vi "MainThang.vi"() -> ()   [LabVIEW 2020]
uses:
  TypeDefs/MainQueueEnumVariant.ctl
  TypeDefs/Item Cluster.ctl
panel:
  in  "Input Buttons":T1
  out "Diplay Array":T2[][](array[typedef])
  out "Dispensing time":dbl format="%.1g"
  out "Dispensing":bool
  out "Amount Returned":string
  out "Amount Deposited":string
  in  "Coin Return":bool
  in  "Deposit":bool
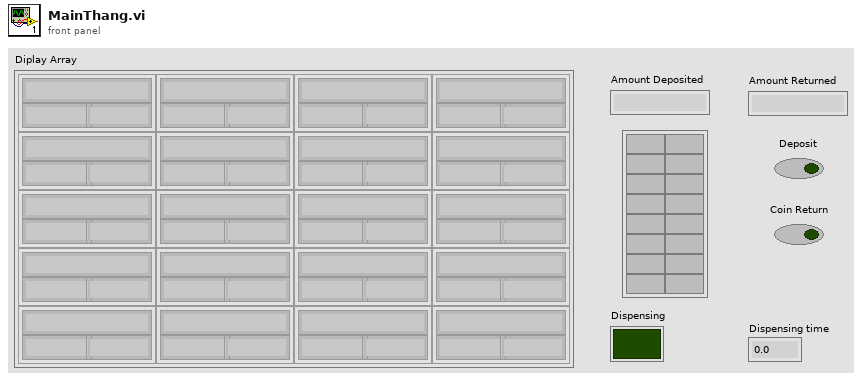
[diagram p1: front panel]
types:
  T1 = cluster{bool, bool, bool, bool, bool, bool, bool, bool, bool, bool, bool, bool, bool, bool, bool, bool}
  T2 = typedef "Item Cluster.ctl" = cluster{"Name":string, "Price":string, "Inventory":string}
  T3 = typedef "MainQueueEnumVariant.ctl" = cluster{enum16{"Init", "Case1", "Case2", "Case3", "Error", "Quit"}, variant}
  T4 = enum16{"Init", "Case1", "Case2", "Case3", "Error", "Quit"}
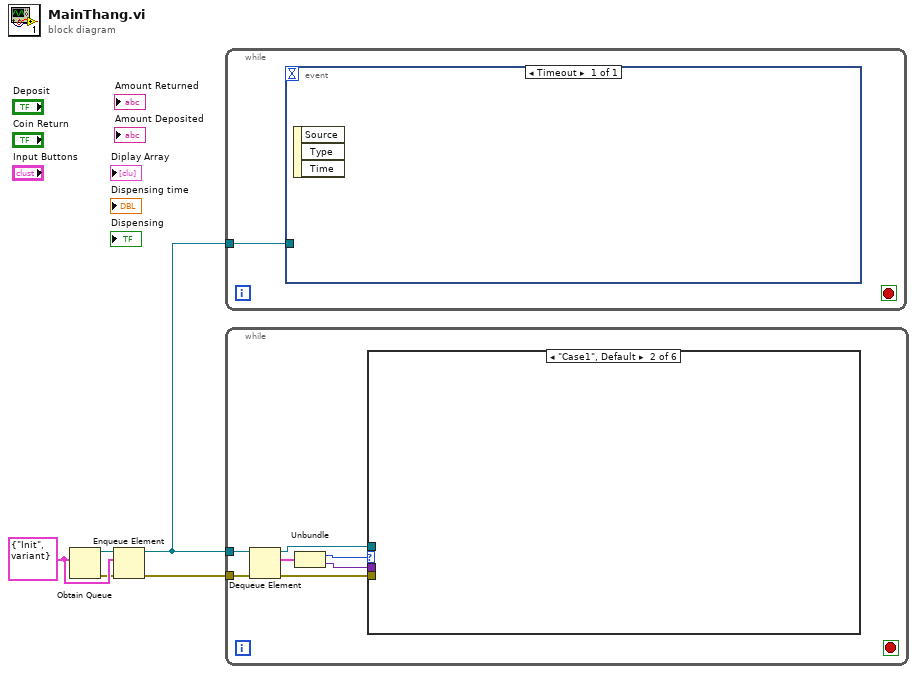
[diagram p0: block diagram]
diagram:
  w5 = T3 {enum."Init", variant}
  n1 = Obtain Queue(element data type=w5) -> (queue out=w4:refnum<queue>, error out=w2:errorcluster)  [unwired: 4 in, 1 out]
  n2 = Enqueue Element(queue=w4, element=w5, error in (no error)=w2) -> (queue out=w3:refnum<queue>, error out=w1:errorcluster)  [unwired: 1 in, 1 out]
  n3 = while {
    tunnel: w3 -> [w6]
    stop <- _ stop-if-true
    n4 = event shown="[0] Timeout" {
      selector: _ -> [_]
      dyn-events: _ -> [_]
      timeout: _ -> [_]
      tunnel: w6 -> [_]
      event Timeout {
        n5 = event-data() -> ()  [unwired: 1 in, 3 out]
      }
    }
  }
  n6 = while {
    tunnel: w3 -> [w13]
    tunnel: w1 -> [w12]
    stop <- _ stop-if-true
    n7 = Dequeue Element(queue=w13, error in (no error)=w12) -> (queue out=w10:refnum<queue>, element=w11:T3, error out=w7:errorcluster)  [unwired: 1 in, 1 out]
    n8 = Unbundle(w11) -> (w9:T4, w8:variant)
    n9 = case shown="\"Case1\", Default" w9 {
      tunnel: w10 -> [_ _ _ _ _ _]
      tunnel: w8 -> [_ _ _ _ _ _]
      tunnel: w7 -> [_ _ _ _ _ _]
      frame "Init" {
      }
      frame "Case1", Default {
      }
      frame "Case2" {
      }
      frame "Case3" {
      }
      frame "Error" {
      }
      frame "Quit" {
      }
    }
  }
